vi "Read Configuration.vi"(7 "Type and Defaults":variant, 8 "error in (no error)":errorcluster, 11 "JSON Config File in":refnum<class "JSON Config File.lvclass">) -> (0 "error out":errorcluster, 2 "Configuration":variant, 3 "JSON Config File out":refnum<class "JSON Config File.lvclass">)   [LabVIEW 2020, in "JSON Config File.lvclass"]
uses:
  JSON Config File.lvclass
  JSON Config File.lvclass/JSON Config File.ctl
  JKI JSON Serialization.lvlib
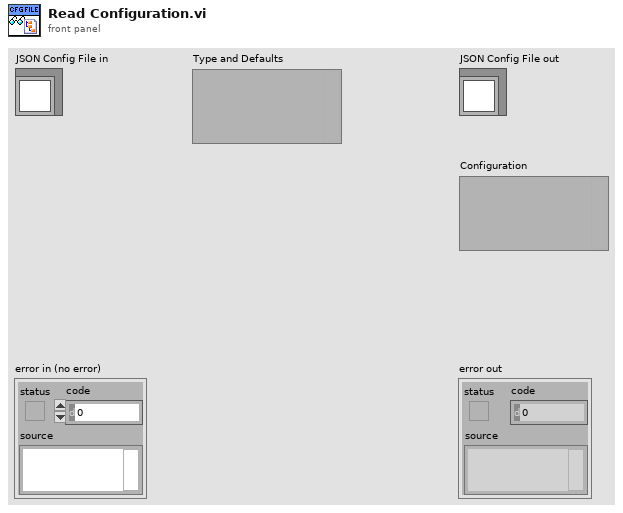
[diagram p1: front panel]
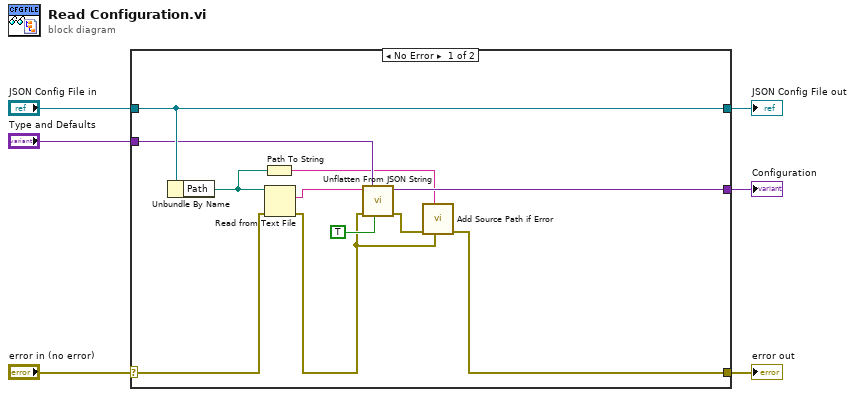
[diagram p0: block diagram]
diagram:
  n1 = case shown="No Error" "error in (no error)" {
    selector: "error in (no error)" -> [w16 w19]
    tunnel: [w7 w19] -> w5
    tunnel: [w17 w18] -> w3
    tunnel: "JSON Config File in" -> [w17 w18]
    tunnel: "Type and Defaults" -> [w14 _]
    tunnel: [w12 _] -> w1
    frame No Error {
      n2 = Unbundle By Name(w17) -> ("Path"=w11:path)
      n3 = Path To String(path=w11) -> (string=w9:string)
      n4 = Read from Text File(file (use dialog)=w11, error in=w16) -> (text=w15:string, error out=w8:errorcluster)  [unwired: 2 in, 2 out]
      n5 = call "Unflatten From JSON String.vi"("Nulls as Defaults (F)"=TRUE, "Type and Defaults"=w14, "error in (no error)"=w8, "JSON String"=w15) -> ("error out"=w10:errorcluster, "Variant"=w12:variant)  [unwired: 6 in]
      n6 = call "Add Source Path if Error.vi"("Upstream Error"=w8, "Source Path or URL"=w9, "error in (no error)"=w10) -> ("error out"=w7:errorcluster)  [unwired: 8 in]
    }
    frame Error {
    }
  }
  "error out" <- w5
  "JSON Config File out" <- w3
  "Configuration" <- w1
